vi "GetScreenSaverEnabled.vi"(8 "error in (no error)":errorcluster, 11 "Engine in":refnum<class "Engine.lvclass">) -> (0 "error out":errorcluster, 2 "Screen Saver Enabled":bool, 3 "Engine out":refnum<class "Engine.lvclass">)   [LabVIEW 2020, in "GLF.lvlib" / "Engine.lvclass"]
uses:
  Engine.lvclass
  Engine.lvclass/Engine.ctl
  <vilib>/Saukko/LV SDL3/Sources/SDL3/Video/Video.lvlib
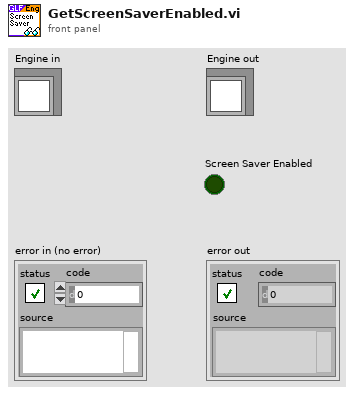
[diagram p1: front panel]
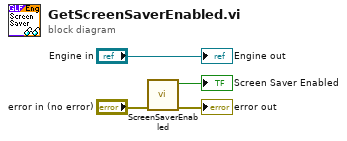
[diagram p0: block diagram]
diagram:
  n1 = call <vilib>:"ScreenSaverEnabled.vi"("No Error"="error in (no error)") -> ("Error Out"=→"error out":errorcluster, "Enabled?"=→"Screen Saver Enabled":bool)  [unwired: 9 in]
  "Engine out" <- "Engine in"
